vi "SendNextStep.vi"(8 "error in (no error)":errorcluster, 10 "StepIndex":u32, 11 "Qbus in":refnum<class "Qbus.lvclass">) -> (0 "error out":errorcluster)   [LabVIEW 2016, in "SeqProcessor.lvlib"]
uses:
  SeqProcessor.lvlib
  <vilib>/addons/Qbus/Qbus.lvclass
  controls/ParallelStep.ctl
  controls/NormalStep.ctl
  controls/StepAction.ctl
  controls/StepResult.ctl
  controls/StepStatus.ctl
  controls/ConditionalStep.ctl
  controls/JumpStep.ctl
  controls/StepIndex.ctl
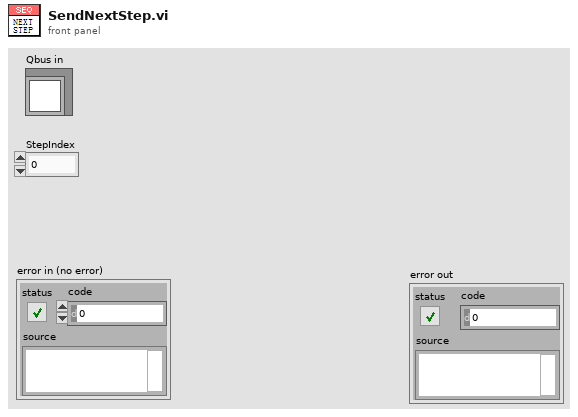
[diagram p1: front panel]
types:
  T1 = typedef "SeqProcessor.lvlib/Step.ctl" = cluster{"Type":T2, "Step":variant}
  T2 = typedef "SeqProcessor.lvlib/StepType.ctl" = enum16{"Normal", "Parallel", "Conditional", "Jump"}
  T3 = typedef "SeqProcessor.lvlib/StepResult.ctl" = cluster{"Status":T4, "Message":string, "Data":variant}
  T4 = typedef "SeqProcessor.lvlib/StepStatus.ctl" = enum16{"Undone", "Finish", "Error"}
  T5 = typedef "SeqProcessor.lvlib/StepIndex.ctl" = cluster{"Index1":u32, "Index2":u32}
  T6 = typedef "SeqProcessor.lvlib/ParallelStep.ctl" = T7[]
  T7 = typedef "SeqProcessor.lvlib/NormalStep.ctl" = cluster{"Action":T8, "Result":T3}
  T8 = typedef "SeqProcessor.lvlib/StepAction.ctl" = cluster{"Action":string, "Process":string, "Data":variant, "Condition":variant}
  T9 = typedef "SeqProcessor.lvlib/ConditionalStep.ctl" = cluster{"Action":T8, "Result":T3}
  T10 = typedef "SeqProcessor.lvlib/JumpStep.ctl" = cluster{"Action":T8, "Jump":i32, "Result":T3}
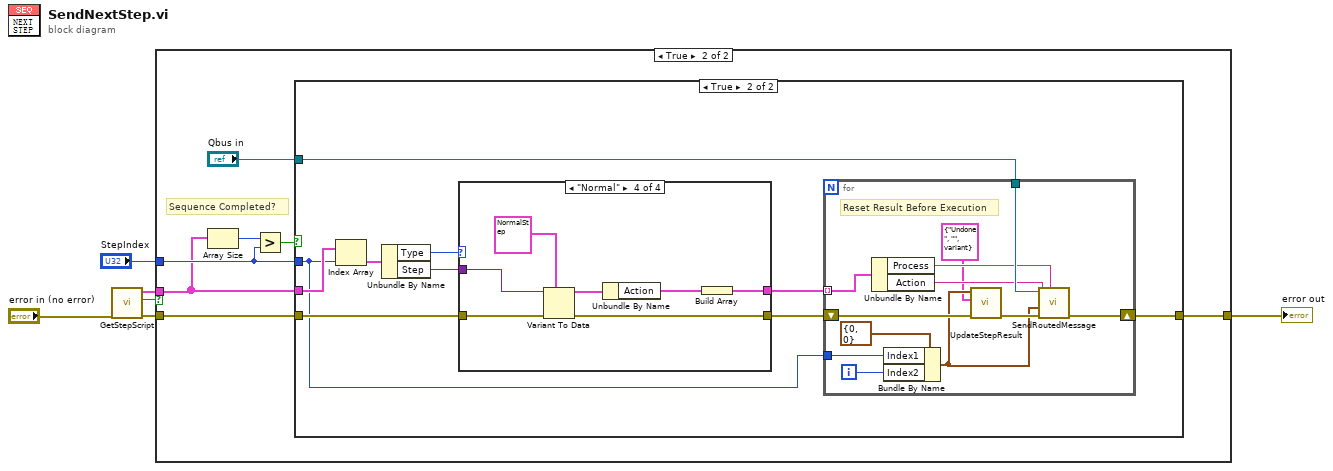
[diagram p0: block diagram]
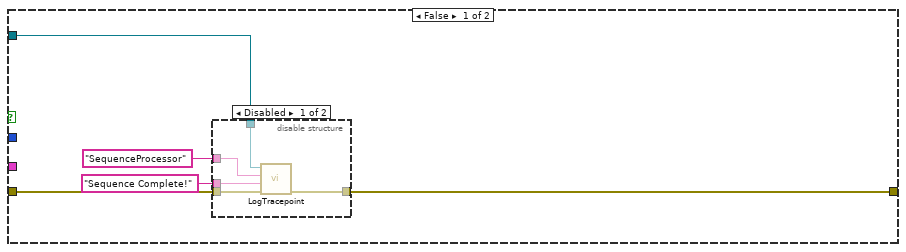
[diagram p3: hidden frame]
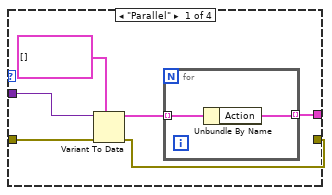
[diagram p5: hidden frame]
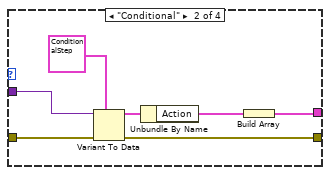
[diagram p6: hidden frame]
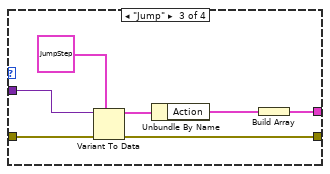
[diagram p7: hidden frame]
diagram:
  n1 = call "GetStepScript.vi"("error in (no error)"="error in (no error)") -> ("error out"=w2:errorcluster, "found"=w3:bool, "StepScript"=w5:T1[])  [unwired: 8 in]
  n2 = case shown="True" w3 {
    tunnel: w5 -> [_ w10]
    tunnel: "StepIndex" -> [_ w13]
    tunnel: w2 -> [w7 w9]
    tunnel: [w7 w8] -> w1
    frame False {
    }
    frame True {
      # "Sequence Completed?"
      n3 = Array Size(array=w10) -> (size(s)=w14:i32)
      n4 = Greater?(x=w14, y=w13) -> (0:w12:bool)
      n5 = case shown="True" w12 {
        tunnel: w13 -> [_ w26]
        tunnel: "Qbus in" -> [w17 w27]
        tunnel: w10 -> [_ w34]
        tunnel: w9 -> [w16 w30]
        tunnel: [w15 w25] -> w8
        frame False {
          n6 = disable-structure shown="Disabled" {
            disable-tunnel: "SequenceProcessor" ("tracepoint") -> [w24 _]
            disable-tunnel: "Sequence Complete!" ("log string") -> [w23 _]
            disable-tunnel: w17 -> [w22 _]
            disable-tunnel: w16 -> [w21 _]
            disable-tunnel: [w20 _] -> w15
            frame Disabled {
              n7 = call "LogTracepoint.vi"("error in (no error)"=w21, "log string"=w23, "tracepoint"=w24, "qbus in"=w22) -> ("error out"=w20:errorcluster)  [unwired: 6 in, 1 out]
            }
            frame Enabled {
            }
          }
        }
        frame True {
          n8 = Index Array(array=w34, index=w26) -> (element=w33:T1)
          n9 = Unbundle By Name(w33) -> ("Type"=w32:T2, "Step"=w31:variant)
          n10 = case shown="\"Normal\"" w32 {
            tunnel: w31 -> [w51 w61 w68 w75]
            tunnel: w30 -> [w50 w60 w67 w74]
            tunnel: [w48 w56 w63 w70] -> w28
            tunnel: [w47 w55 w62 w69] -> w29
            frame "Parallel" {
              n11 = Variant To Data(error in=w50, type=T6 [] ("ParallelStep"), Variant=w51) -> (data=w49:T6, error out=w47:errorcluster)
              n12 = for {
                tunnel: w49 -> [w54] mode=indexing
                tunnel: [w53] -> w48 mode=indexing
                n13 = Unbundle By Name(w54) -> ("Action"=w53:T8)
              }
            }
            frame "Conditional" {
              n14 = Variant To Data(error in=w60, type=T9 {"Action"={"Action"="", "Process"="", "Data"=variant, "Condition"=variant(bool FALSE)}, "Result"={"Status"=enum."Undone", "Message"="", "Data"=variant}} ("ConditionlStep"), Variant=w61) -> (data=w58:T9, error out=w55:errorcluster)
              n15 = Unbundle By Name(w58) -> ("Action"=w57:T8)
              n16 = Build Array(w57) -> (w56:T8[])
            }
            frame "Jump" {
              n17 = Variant To Data(error in=w67, type=T10 {"Action"={"Action"="", "Process"="", "Data"=variant, "Condition"=variant(bool FALSE)}, "Jump"=0, "Result"={"Status"=enum."Undone", "Message"="", "Data"=variant}} ("JumplStep"), Variant=w68) -> (data=w66:T10, error out=w62:errorcluster)
              n18 = Unbundle By Name(w66) -> ("Action"=w64:T8)
              n19 = Build Array(w64) -> (w63:T8[])
            }
            frame "Normal" {
              n20 = Variant To Data(error in=w74, type=T7 {"Action"={"Action"="", "Process"="", "Data"=variant, "Condition"=variant(bool FALSE)}, "Result"={"Status"=enum."Undone", "Message"="", "Data"=variant}} ("NormalStep"), Variant=w75) -> (data=w73:T7, error out=w69:errorcluster)
              n21 = Unbundle By Name(w73) -> ("Action"=w71:T8)
              n22 = Build Array(w71) -> (w70:T8[])
            }
          }
          n23 = for {
            tunnel: w28 -> [w45] mode=indexing
            tunnel: w27 -> [w46]
            tunnel: w26 -> [w41]
            shift-right: [w39] -> w25
            shift-left: w29 -> [w38]
            i -> [w40]
            # "Reset Result Before Execution"
            n24 = Unbundle By Name(w45) -> ("Process"=w44:string, "Action"=w43:string)
            n25 = Bundle By Name(cluster=T5 {"Index1"=0, "Index2"=0} ("Index"), "Index1"=w41, "Index2"=w40) -> (w36:T5)
            n26 = call "UpdateStepResult.vi"("error in (no error)"=w38, "Result"=T3 {"Status"=enum."Undone", "Message"="", "Data"=variant}, "Index"=w36) -> ("error out"=w37:errorcluster)  [unwired: 7 in, 1 out]
            n27 = call <vilib>:"SendRoutedMessage.vi"("listener process"=w44, "error in (no error)"=w37, "message value"=w36, "message name"=w43, "Qbus in"=w46) -> ("error in (no error)"=w39:errorcluster)  [unwired: 5 in, 1 out]
          }
        }
      }
    }
  }
  "error out" <- w1
